vi "VisionDrive.vi"(9 "RightMotorInput":dbl, 10 "LeftMotorInput":dbl) -> (1 "RightMotorOutput":dbl, 2 "LeftMotorOutput":dbl)   [LabVIEW 2015]
uses:
  Utilities/GlobalVisionVars.vi
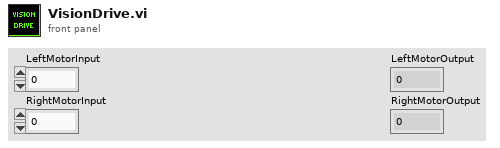
[diagram p1: front panel]
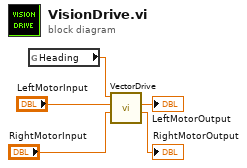
[diagram p0: block diagram]
diagram:
  n1 = global read "GlobalVisionVars.vi" "Heading"() -> (w5:dbl)
  n2 = call "VectorDrive.vi"("RightMotorInput"="RightMotorInput", "LeftMotorInput"="LeftMotorInput", "setpoint"=w5) -> ("RightMotorOutput"=→"RightMotorOutput":dbl, "LeftMotorOutput"=→"LeftMotorOutput":dbl)  [unwired: 7 in]
